vi "ckDts.vi"(5 "rdDts":string, 9 "rdMatch":string) -> (6 "OK":bool, 10 "dataOut":string)   [LabVIEW 2015]
panel:
  out "match":bool
  out "crc":string
  out "calCRC":string
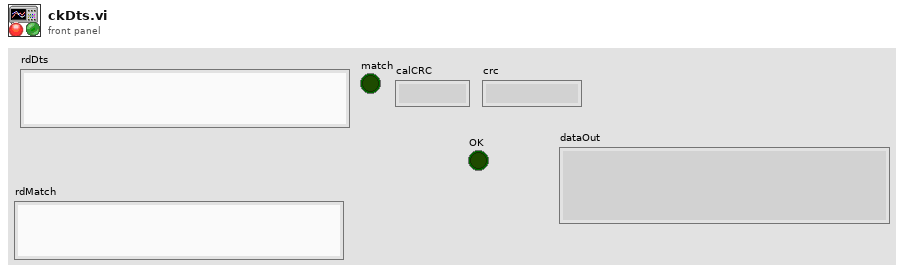
[diagram p1: front panel]
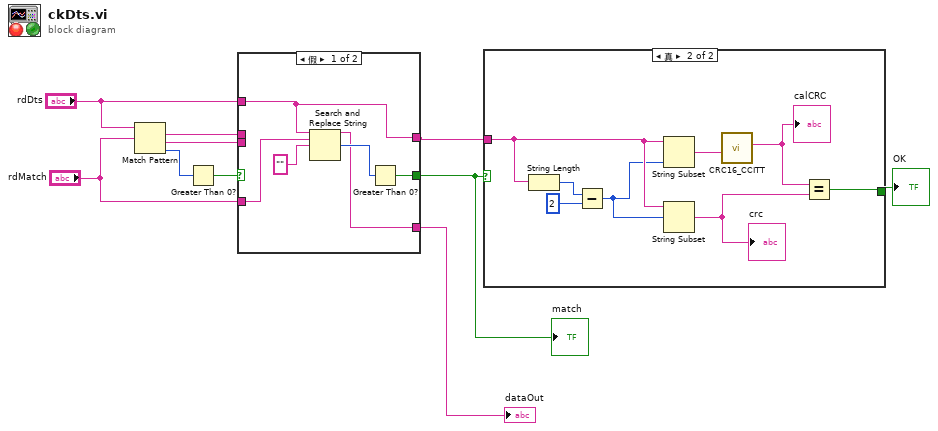
[diagram p0: block diagram]
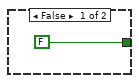
[diagram p2: hidden frame]
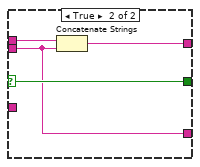
[diagram p3: hidden frame]
diagram:
  n1 = Match Pattern(string="rdDts", regular expression="rdMatch") -> (match substring=w9:string, after substring=w8:string, offset past match=w10:i32)  [unwired: 1 in, 1 out]
  n2 = Greater Than 0?(x=w10) -> (x > 0?=w5:bool)
  n3 = case shown="假" w5 {
    selector: w5 -> [_ w18]
    tunnel: w9 -> [_ w20]
    tunnel: w8 -> [_ w17]
    tunnel: "rdDts" -> [w14 _]
    tunnel: "rdMatch" -> [w15 _]
    tunnel: [w14 w19] -> w3
    tunnel: [w12 w18] -> w4
    tunnel: [w11 w17] -> w1
    frame False {
      n4 = Search and Replace String(input string=w14, search string=w15, replace string="" ("替换字符串(\"\")")) -> (result string=w11:string, number of replacements=w13:i32)  [unwired: 5 in, 2 out]
      n5 = Greater Than 0?(x=w13) -> (x > 0?=w12:bool)
    }
    frame True {
      n6 = Concatenate Strings(w20, w17) -> (w19:string)
    }
  }
  "match" <- w4
  "dataOut" <- w1
  n7 = case shown="真" w4 {
    tunnel: w3 -> [_ w24]
    tunnel: [FALSE w23] -> w2
    frame False {
    }
    frame True {
      n8 = String Length(string=w24) -> (length=w29:i32)
      n9 = Subtract(x=w29, y=2) -> (x-y=w22:i32)
      n10 = String Subset(string=w24, length (rest)=w22) -> (substring=w27:string)  [unwired: 1 in]
      n11 = String Subset(string=w24, offset (0)=w22) -> (substring=w26:string)  [unwired: 1 in]
      "crc" <- w26
      n12 = call "CRC16_CCITT.vi"("sDt"=w27) -> ("CRC16_LH"=w25:string)  [unwired: 8 in, 2 out]
      "calCRC" <- w25
      n13 = Equal?(x=w25, y=w26) -> (x = y?=w23:bool)
    }
  }
  "OK" <- w2
